vi "Project Configure UI.vi"(8 "error in (no error)":errorcluster, 10 "Project In":refnum<class "Project.lvclass">, 11 "SerializableObject in":refnum<class>) -> (0 "error out":errorcluster, 3 "SerializableObject out":refnum<class>)   [LabVIEW 2015, in "Project.lvclass"]
uses:
  Project.lvclass
  RUN_MODE_TYPEDEF.ctl
  Project Configure UI State.ctl
  Project.lvclass/Project.ctl
  <vilib>/Utility/miscctls.llb/LVRowAndColumnTypeDef.ctl
  Editor/Editor.lvclass
panel:
  in  "UI Title":string
  in  "Stop If Fail":bool
  in  "Stop If Error":bool
  in  "Run Mode":T1
  in  "Layout":T2={"Order"=enum."LeftRight", "Row"=2, "Column"=2, "Margin"=5}
  in  "Config File":string
  in  "Variable Tree":string(tree)
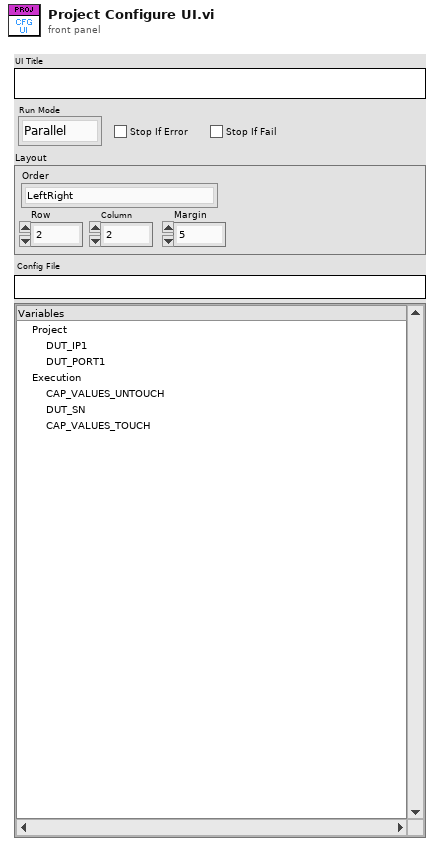
[diagram p1: front panel]
types:
  T1 = typedef "Project.lvclass/RUN_MODE_TYPEDEF.ctl" = enum16{"Parallel", "Batch"}
  T2 = cluster{"Order":enum16{"LeftRight", "TopDown"}, "Row":i32, "Column":i32, "Margin":i32}
  T3 = cluster{"Operation":string, "Tag":string, "Current Name":string, "New Name":string}
  T4 = typedef "Project.lvclass/Project Configure UI State.ctl" = enum16{"VAR_RENAME", "VAR_OP", "UI_LOOP", "INIT", "END"}
  T5 = typedef "LVRowAndColumnTypeDef.ctl" = cluster{"Row":i32, "Column":i32}
  T6 = typedef "UI_CONFIG_TYPEDEF.ctl" = cluster{"Title":string, "Layout":cluster{"Order":enum16{"LeftRight", "TopDown"}, "Row":i32, "Column":i32, "Margin":i32}}
  T7 = typedef "LVPoint32TypeDef.ctl" = cluster{"Horizontal":i32, "Vertical":i32}
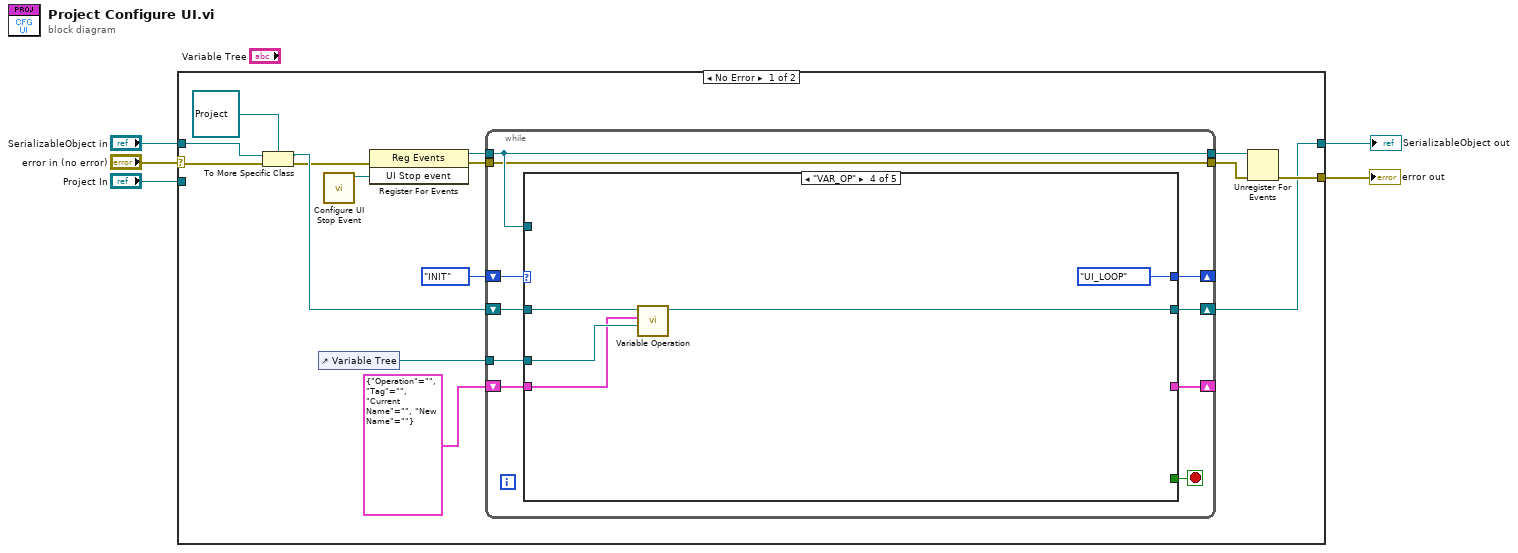
[diagram p0: block diagram]
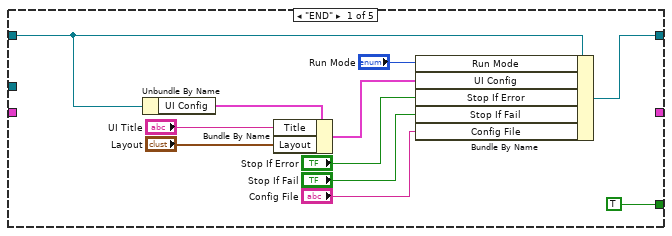
[diagram p2: hidden frame]
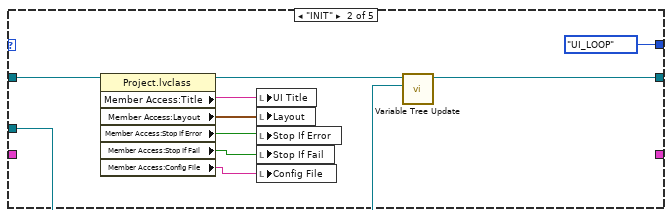
[diagram p3: hidden frame]
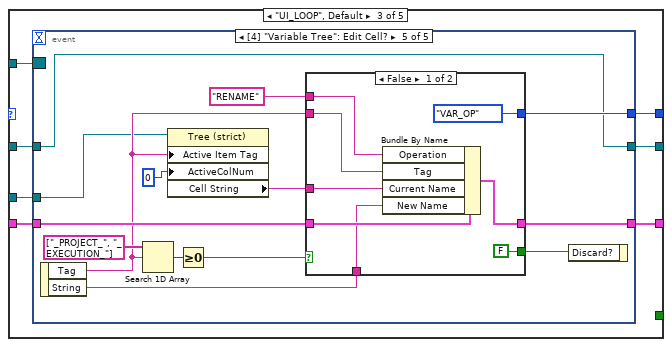
[diagram p4: hidden frame]
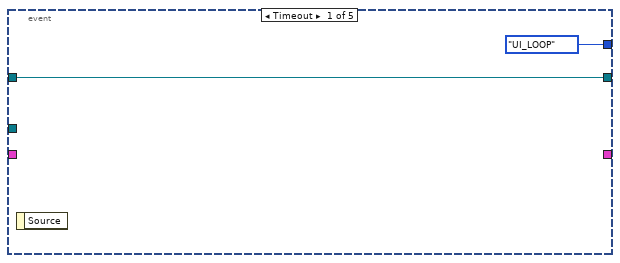
[diagram p5: hidden frame]
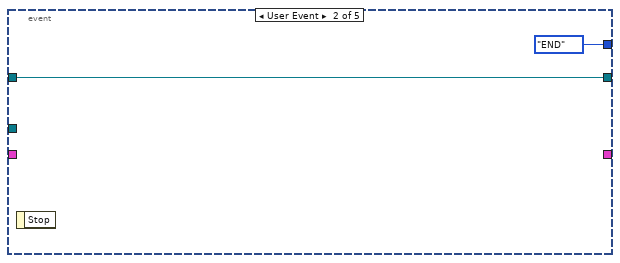
[diagram p6: hidden frame]
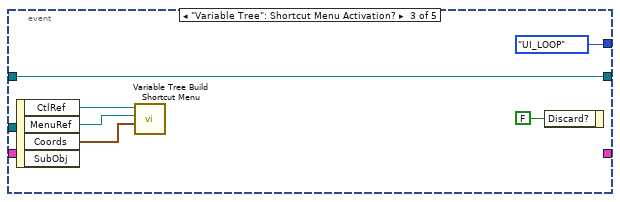
[diagram p7: hidden frame]
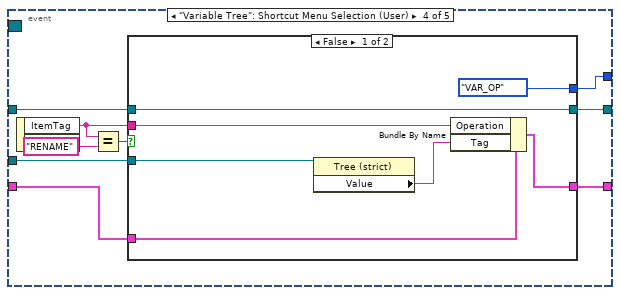
[diagram p8: hidden frame]
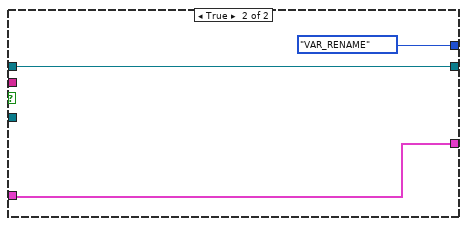
[diagram p9: hidden frame]
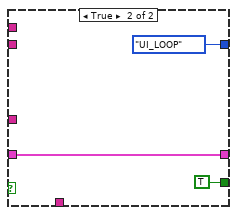
[diagram p10: hidden frame]
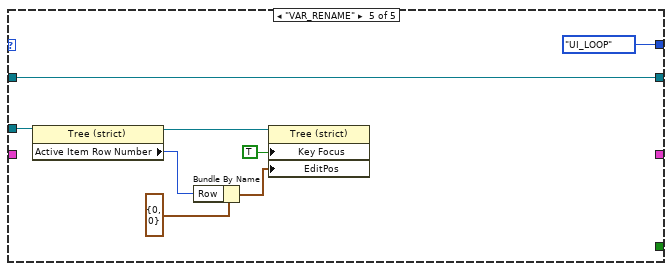
[diagram p11: hidden frame]
diagram:
  n1 = case shown="No Error" "error in (no error)" {
    selector: "error in (no error)" -> [w13 w127]
    tunnel: [w15 w127] -> w4
    tunnel: "SerializableObject in" -> [w20 w126]
    tunnel: [w12 w126] -> w2
    tunnel: "Project In" -> [_ _]
    frame No Error {
      n2 = To More Specific Class(target class=refnum<class "Project.lvclass"> refnum ("Project.lvclass"), reference=w20, error in=w13) -> (specific class reference=w9:refnum<class "Project.lvclass">, error out=w8:errorcluster)
      n3 = control-ref of="Variable Tree"() -> (w6:refnum<vi>)
      n4 = call "Configure UI Stop Event.vi"() -> ("UI Stop event"=w10:refnum<user-event>)  [unwired: 11 in]
      n5 = register-events(error in=w8, w10) -> (reference out=w19:refnum<event-registration>, error out=w17:errorcluster)  [unwired: 1 in]
      n6 = while {
        tunnel: w19 -> [w30]
        tunnel: [w30] -> w18
        tunnel: w17 -> [w29]
        tunnel: [w29] -> w16
        shift-right: [w27] -> w12
        shift-left: w9 -> [w28]
        shift-right: [w25] -> _
        shift-left: Project_Configure_UI_State."INIT" -> [w26]
        tunnel: w6 -> [w23]
        shift-right: [w22] -> _
        shift-left: T3 {"Operation"="", "Tag"="", "Current Name"="", "New Name"=""} -> [w21]
        stop <- w24 stop-if-true
        n7 = case shown="\"VAR_OP\"" w26 {
          tunnel: w30 -> [_ _ w58 _ _]
          tunnel: w28 -> [w35 w50 w57 w116 w124]
          tunnel: [w34 w46 w56 w115 w124] -> w27
          tunnel: [_ Project_Configure_UI_State."UI_LOOP" w54 Project_Configure_UI_State."UI_LOOP" Project_Configure_UI_State."UI_LOOP"] -> w25
          tunnel: [TRUE _ _ _ _] -> w24
          tunnel: w23 -> [_ w45 w55 w114 w123]
          tunnel: [_ _ w53 _ _] -> w22
          tunnel: w21 -> [_ _ w52 w113 _]
          frame "END" {
            n8 = Unbundle By Name(w35) -> ("UI Config"=w39:T6)
            n9 = Bundle By Name(cluster=w39, "Title"="UI Title", "Layout"="Layout") -> (w38:T6)
            n10 = Bundle By Name(cluster=w35, "Run Mode"="Run Mode", "UI Config"=w38, "Stop If Error"="Stop If Error", "Stop If Fail"="Stop If Fail", "Config File"="Config File") -> (w34:refnum<class "Project.lvclass">)
          }
          frame "INIT" {
            n11 = property class="Project.lvclass"(reference=w50) -> (reference out=w47:refnum<class "Project.lvclass">, "Member Access:Title"=w49:string, "Member Access:Layout"=w48:T2, "Member Access:Stop If Error"=w44:bool, "Member Access:Stop If Fail"=w43:bool, "Member Access:Config File"=w42:string)  [unwired: 1 in, 1 out]
            n12 = local write "UI Title"(w49) -> ()
            n13 = local write "Layout"(w48) -> ()
            n14 = local write "Stop If Error"(w44) -> ()
            n15 = local write "Stop If Fail"(w43) -> ()
            n16 = local write "Config File"(w42) -> ()
            n17 = call "Variable Tree Update .vi"("Variable Tree"=w45, "Project in"=w47) -> ("Project out"=w46:refnum<class "Project.lvclass">)  [unwired: 8 in, 1 out]
          }
          frame "UI_LOOP", Default {
            n18 = event shown="[4] \"Variable Tree\": Edit Cell?" {
              selector: w58 -> [_ _ _ _ _]
              dyn-events: _ -> [_ _ _ _ _]
              timeout: _ -> [_ _ _ _ _]
              tunnel: w57 -> [w60 w62 w68 w77 w92]
              tunnel: [w60 w62 w68 w76 w92] -> w56
              tunnel: [Project_Configure_UI_State."UI_LOOP" Project_Configure_UI_State."END" Project_Configure_UI_State."UI_LOOP" w69 w94] -> w54
              tunnel: w55 -> [_ _ _ w72 w88]
              tunnel: [_ _ _ w70 w95] -> w53
              tunnel: w52 -> [_ _ _ w71 w97]
              event Timeout {
                n19 = event-data() -> ()  [unwired: 1 in, 1 out]
              }
              event User Event {
                n20 = event-data() -> ()  [unwired: 1 in, 1 out]
              }
              event "Variable Tree": Shortcut Menu Activation? {
                n21 = event-data() -> ("CtlRef"=w67:refnum<vi>, "MenuRef"=w66:refnum<k9>, "Coords"=w65:T7)  [unwired: 1 in, 1 out]
                n22 = call "Variable Tree Build Shortcut Menu.vi"("Coords"=w65, "MenuRef"=w66, "Variable Tree"=w67) -> ()  [unwired: 8 in, 1 out]
                n23 = event-data("Discard?"=FALSE) -> ()  [unwired: 1 in, 1 out]
              }
              event "Variable Tree": Shortcut Menu Selection (User) {
                n24 = event-data() -> ("ItemTag"=w75:string)  [unwired: 1 in, 1 out]
                n25 = Equal?(x=w75, y="RENAME") -> (x = y?=w73:bool)
                n26 = case shown="False" w73 {
                  tunnel: w77 -> [w84 w87]
                  tunnel: [w84 w87] -> w76
                  tunnel: w72 -> [w79 _]
                  tunnel: w75 -> [w81 _]
                  tunnel: [Project_Configure_UI_State."VAR_OP" Project_Configure_UI_State."VAR_RENAME"] -> w69
                  tunnel: w71 -> [w82 w85]
                  tunnel: [w80 w85] -> w70
                  frame False {
                    n27 = property class="Tree (strict)"(reference=w79) -> ("Value"=w78:string)  [unwired: 1 in, 2 out]
                    n28 = Bundle By Name(cluster=w82, "Operation"=w81, "Tag"=w78) -> (w80:T3)
                  }
                  frame True {
                  }
                }
              }
              event "Variable Tree": Edit Cell? {
                n29 = event-data() -> ("Tag"=w89:string, "String"=w99:string)  [unwired: 1 in]
                n30 = Search 1D Array(1D array=string[] ["_PROJECT_", "_EXECUTION_"], element=w89) -> (index of element=w100:i32)  [unwired: 1 in]
                n31 = property class="Tree (strict)"(reference=w88, "Active Item Tag"=w89, "ActiveColNum"=0 ("Active Cell:Active Column Number")) -> ("Cell String"=w90:string)  [unwired: 1 in, 2 out]
                n32 = Greater Or Equal To 0?(x=w100) -> (x >= 0?=w98:bool)
                n33 = case shown="False" w98 {
                  tunnel: w99 -> [w108 _]
                  tunnel: w97 -> [w109 w112]
                  tunnel: "RENAME" ("Operation") -> [w103 _]
                  tunnel: [w107 w112] -> w95
                  tunnel: [Project_Configure_UI_State."VAR_OP" Project_Configure_UI_State."UI_LOOP"] -> w94
                  tunnel: [FALSE TRUE] -> w93
                  tunnel: w90 -> [w104 _]
                  tunnel: w89 -> [w102 _]
                  frame False {
                    n34 = Bundle By Name(cluster=w109, "Operation"=w103, "Tag"=w102, "Current Name"=w104, "New Name"=w108) -> (w107:T3)
                  }
                  frame True {
                  }
                }
                n35 = event-data("Discard?"=w93) -> ()  [unwired: 1 in, 1 out]
              }
            }
          }
          frame "VAR_OP" {
            n36 = call "Variable Operation.vi"("Variable Tree"=w114, "Variable Data"=w113, "Project in"=w116) -> ("Project out"=w115:refnum<class "Project.lvclass">)  [unwired: 6 in, 2 out]
          }
          frame "VAR_RENAME" {
            n37 = property class="Tree (strict)"(reference=w123) -> (reference out=w122:refnum<vi>, "Active Item Row Number"=w120:i32)  [unwired: 1 in, 1 out]
            n38 = Bundle By Name(cluster=T5 {"Row"=0, "Column"=0} ("Edit Position"), "Row"=w120) -> (w118:T5)
            n39 = property class="Tree (strict)"(reference=w122, "Key Focus"=TRUE, "EditPos"=w118) -> ()  [unwired: 1 in, 2 out]
          }
        }
      }
      n40 = Unregister For Events(event registration refnum=w18, error in=w16) -> (error out=w15:errorcluster)
    }
    frame Error {
    }
  }
  "error out" <- w4
  "SerializableObject out" <- w2
